vi "mqttCmdQOSread.vi"(0 "mqttBrokerCommand in":refnum<class "mqttCmd.lvclass">, 11 "error in (no error)":errorcluster) -> (4 "mqttBrokerCommand out":refnum<class "mqttCmd.lvclass">, 6 "QoS":T1, 15 "error out":errorcluster)   [LabVIEW 2014, in "labview-mqtt.lvlib" / "mqttCmd.lvclass"]
uses:
  mqttCmd.lvclass
  mqttTypedef/mqttQOSlevel.ctl
  mqttCmd.lvclass/mqttCmd.ctl
  labview-mqtt.lvlib
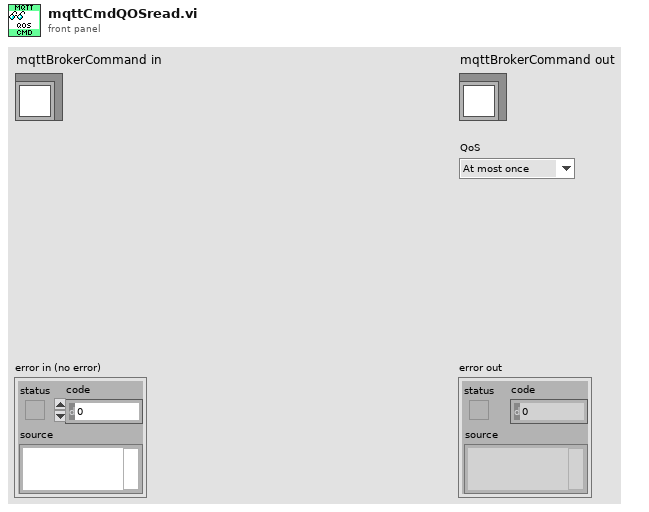
[diagram p1: front panel]
types:
  T1 = typedef "labview-mqtt.lvlib/mqttQOSlevel.ctl" = enum8{"At most once", "At least once", "Exactly once", "Reserved"}
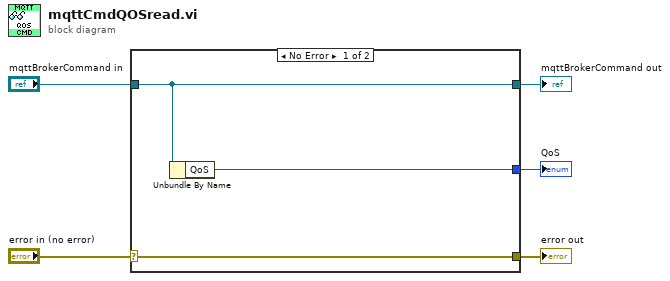
[diagram p0: block diagram]
diagram:
  n1 = case shown="No Error" "error in (no error)" {
    selector: "error in (no error)" -> [w8 w9]
    tunnel: [w8 w9] -> w4
    tunnel: [w7 w10] -> w2
    tunnel: "mqttBrokerCommand in" -> [w7 w10]
    tunnel: [w6 _] -> w1
    frame No Error {
      n2 = Unbundle By Name(w7) -> ("QoS"=w6:T1)
    }
    frame Error {
    }
  }
  "error out" <- w4
  "mqttBrokerCommand out" <- w2
  "QoS" <- w1
